vi "Set Error.vi"(10 "Error":errorcluster, 11 "jettl in":refnum<class "jettl.lvclass">) -> (3 "jettl out":refnum<class "jettl.lvclass">)   [LabVIEW 2021, in "jettl.lvlib" / "jettl.lvclass"]
uses:
  jettl.lvclass
  jettl.lvclass/jettl.ctl
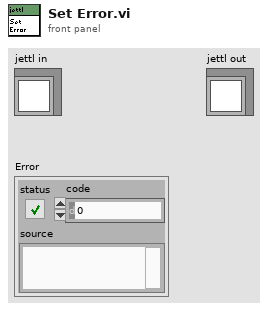
[diagram p1: front panel]
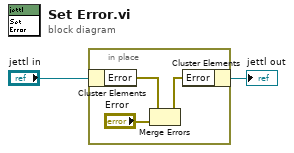
[diagram p0: block diagram]
diagram:
  n1 = in-place {
    n2 = in-place-cluster #1("jettl in") -> ("Error"=w5:errorcluster)
    n3 = Merge Errors(w5, "Error") -> (w4:errorcluster)
    n4 = in-place-cluster #1("Error"=w4) -> (→"jettl out":refnum<class "jettl.lvclass">)
  }
